vi "SR430.set bins per record.vi"(0 "i ref in":refnum<vi>, 2 "binsPerRecord":i32, 3 "ms timeout (10000)":i32=10000, 5 "error in (no error)":errorcluster) -> (14 "i ref out":refnum<vi>, 16 "actBinsPerRecored":i32, 17 "timed out":bool, 19 "error out":errorcluster)   [LabVIEW 2014, in "SR430.lvlib"]
doc: "Sets the bins per record at the SR430. The record length at the instrument ranges from 1024 bins to 16384 bins in steps of 1024 bins. The valid range for this class is from 1 to 16384 bins. The value set at the instrument equals the input value that will be rounded to the next higher step of 1024 bins at the instrument. However, the value used by this class when reading the value equals exactly the input value by truncating the data delivered by the instrument.\n\nExample 1: The input value is 1024 bins, the value at the instrument will be 1024 and the data will have exactly 384 bins.\n\nExample 2: The input value is 384, the value at the instrument will be 1024 but the data will be truncated to exactly 384 bins."
uses:
  SR430.lvlib
  CS_Core/CSApplicationBaseClasses/MCSBase/MCSBase.directionType.ctl
  CS_Core/CSApplicationBaseClasses/MCSBase/MCSBase.serviceType.ctl
  CSlibraries/UtilityLib/UtilityLib.valueStatus.ctl
  CS_Core/CSSystem/CoreDefs/CoreDefs.error_type.ctl
  instr.lib/SR430/SR430Driver.lvlib
  CS_Core/CSSystem/CoreLib/CoreLib.lvlib
  CS_Core/CSApplicationBaseClasses/MCSBase/MCSBase.lvlib
  CSlibraries/UtilityLib/UtilityLib.lvlib
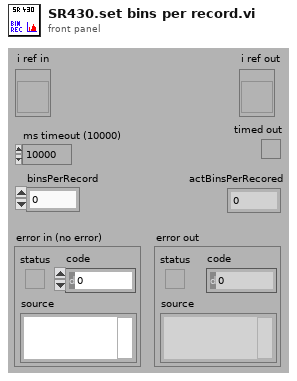
[diagram p1: front panel]
types:
  T1 = typedef "UtilityLib.lvlib/UtilityLib.valueStatus.ctl" = enum16{"no info available", "stand by/off", "on", "warning", "alarm/malfunction", "not implemented", "user action required", "important information", "system default", "control default", "indicator default", "button default"}
  T2 = typedef "MCSBase.lvlib/MCSBase.serviceType.ctl" = enum16{"counts", "totalCounts", "binWidth", "nOfBins", "nOfRecords", "status", "discrLevel", "discrSlope", "triggerLevel", "triggerSlope"}
  T3 = typedef "MCSBase.lvlib/MCSBase.directionType.ctl" = enum16{"unknown", "update actual value", "update nominal value", "update both"}
  T4 = typedef "CoreDefs.error_type.ctl" = enum16{"no error", "can't load process", "can't unload process", "process does not exist", "can't install process", "can't remove process", "unknown function", "time out", "can't execute function", "duplicate queue name", "super not found", "caller queue invalid", "can't ping process", "unknown error", "VISA Error", "VISA timeout", "GPIB timeout", "GPIB error", "communication error", "data type mismatch", "can't read data from OPC server", "can't write data to OPC server", "OET error", "function not implemented", "process already exists", "invalid Shared Variable name", "error writing Shared Variable", "error reading Shared Variable", "invalid client name", "corrupt database", "unknown class", "call not authorized", "parameter out of range", "OET timeout: can't get data to modify", "invalid queue name", "requested operation incompatible with current state", "event undefined", "event disabled", "state undefined", "caller is not a friend", "EventBuilder: bad eventID", "EventBuilder: no DAQ devices", "a thread must not stop itself", "UNUSED ELEMENT4", "DiscArchiver: eventData incomplete", "DiscArchiver: eventData does not belong to run", "DiscArchiver: can't open file", "DiscArchiver: can't write to file", "DiscArchiver: available disc space low", "can't acquire semaphore", "error reading data from database", "notifier object is not existing", "can't register process", "can't unregister process", "illegal event type", "object disabled", "object already exists", "can't change state", "Instrument not found", "no connection to remote node", "invalid reference", "N/A", "UNUSED ELEMENT 1", "element not found", "illegal TCP/IP connection detected", "object does not exist", "invalid access ID", "unknown CS system", "invalid privilige", "unsupported data type", "unsupported server type", "IO server already exists", "Shared Variable already exists"}
  T5 = typedef "SR430Driver.lvlib/SR430_VISA Control.ctl" = cluster{"VISA resource name":refnum<visa-resource-name>}
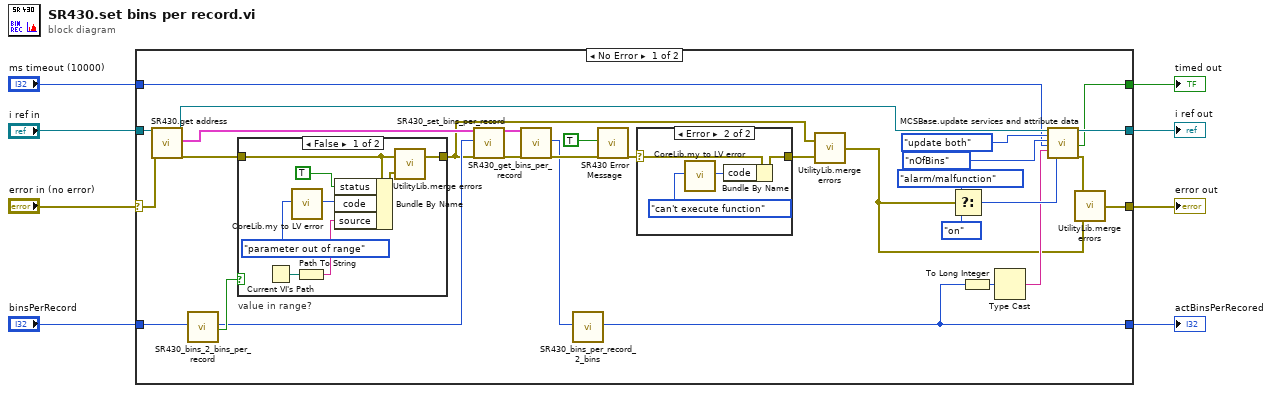
[diagram p0: block diagram]
diagram:
  n1 = case shown="No Error" "error in (no error)" {
    selector: "error in (no error)" -> [w35 w53]
    tunnel: "i ref in" -> [w38 w54]
    tunnel: "binsPerRecord" -> [w36 _]
    tunnel: [w13 _] -> w6
    tunnel: [w16 w54] -> w5
    tunnel: [w14 w53] -> w4
    tunnel: "ms timeout (10000)" -> [w10 _]
    tunnel: [w9 _] -> w2
    frame No Error {
      n2 = call "SR430.get address.vi"("i ref in"=w38, "error in (no error)"=w35) -> ("i ref out"=w11:refnum<vi>, "address"=w37:T5, "error out"=w34:errorcluster)  [unwired: 15 in]
      n3 = call "SR430_bins_2_bins_per_record.vi"("bins"=w36) -> ("binPerRecord"=w31:i32, "In Range?"=w32:bool)  [unwired: 16 in, 1 out]
      n4 = case "value in range?" shown="False" w32 {
        tunnel: [w45 w47] -> w24
        tunnel: w34 -> [w40 w47]
        frame False {
          n5 = Current VI's Path() -> (path=w42:path)
          n6 = call "CoreLib.my to LV error.vi"("ErrorTypes"=CoreDefs.error_type."parameter out of range") -> ("LV error code"=w44:i32)  [unwired: 17 in, 1 out]
          n7 = Path To String(path=w42) -> (string=w41:string)
          n8 = Bundle By Name(cluster=w40, "status"=TRUE, "code"=w44, "source"=w41) -> (w39:errorcluster)
          n9 = call "UtilityLib.merge errors.vi"("error2 (no error)"=w39, "error1 (no error)"=w40) -> ("error out"=w45:errorcluster)
        }
        frame True {
        }
      }
      n10 = call "SR430_set_bins_per_record.vi"("address"=w37, "binsPerRecord"=w31, "error in (no error)"=w24) -> ("address out"=w29:T5, "error out"=w30:errorcluster)  [unwired: 15 in]
      n11 = call "SR430_get_bins_per_record.vi"("address"=w29, "error in (no error)"=w30) -> ("binsPerRecord"=w27:i32, "error out"=w28:errorcluster)  [unwired: 15 in, 1 out]
      n12 = call "SR430_bins_per_record_2_bins.vi"("binsPerRecord"=w27) -> ("bins"=w13:i32)  [unwired: 16 in, 2 out]
      n13 = call "SR430 Error Message.vi"("addMessageToSource"=TRUE ("add message to source"), "error in (no error)"=w28) -> ("error out"=w33:errorcluster)  [unwired: 14 in, 3 out]
      n14 = case shown="Error" w33 {
        selector: w33 -> [w48 w52]
        tunnel: [w48 w49] -> w25
        frame No Error {
        }
        frame Error {
          n15 = call "CoreLib.my to LV error.vi"("ErrorTypes"=CoreDefs.error_type."can't execute function") -> ("LV error code"=w51:i32)  [unwired: 17 in, 1 out]
          n16 = Bundle By Name(cluster=w52, "code"=w51) -> (w49:errorcluster)
        }
      }
      n17 = call "UtilityLib.merge errors.vi"("error2 (no error)"=w25, "error1 (no error)"=w24) -> ("error out"=w15:errorcluster)
      n18 = Select(t=UtilityLib.valueStatus."alarm/malfunction", s=w15, f=UtilityLib.valueStatus."on" ("quality")) -> (s? t:f=w22:T1)
      n19 = To Long Integer(number=w13) -> (32bit integer=w12:i32)
      n20 = Type Cast(x=w12) -> (*(type *) &x=w19:string)  [unwired: 1 in]
      n21 = call "MCSBase.update services and attribute data.vi"("i ref in"=w11, "direction"=MCSBase.directionType."update both", "service"=MCSBase.serviceType."nOfBins", "ms timeout (10000)"=w10, "value"=w19, "quality"=w22) -> ("i ref out"=w16:refnum<vi>, "timed out"=w9:bool, "error out"=w23:errorcluster)  [unwired: 11 in]
      n22 = call "UtilityLib.merge errors.vi"("error2 (no error)"=w15, "error1 (no error)"=w23) -> ("error out"=w14:errorcluster)
    }
    frame Error {
    }
  }
  "error out" <- w4
  "i ref out" <- w5
  "timed out" <- w2
  "actBinsPerRecored" <- w6
